vi "get_mlt.vi"   [LabVIEW 2012]
uses:
  <vilib>/addons/internet/NI_InternetTK_Core_VIs.lvlib
types:
  T1 = typedef "CGI Connection Info.ctl" = cluster{"name":string, "type":T2, "session":T3}
  T2 = typedef "CGI Request Type.ctl" = enum16{"cgi", ".spool first", ".spool", ".spool last"}
  T3 = typedef "HTTP Session.ctl" = refnum<k1>
  T4 = typedef "NI_FTP.lvlib/Keyed Array.ctl" = cluster{"keys":string[], "values":string[]}
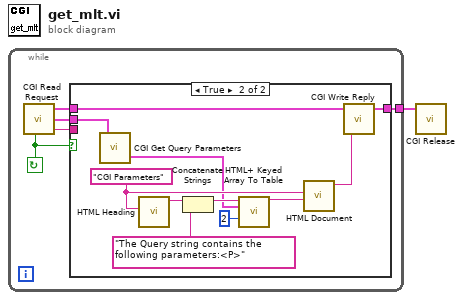
[diagram p0: block diagram]
diagram:
  n1 = while {
    tunnel: [w5] -> w1
    stop <- w4 continue-if-true
    n2 = call <vilib>:"CGI Read Request.vi"() -> ("valid request?"=w4:bool, "cgi connection info"=w6:T1, "env"=w3:T4, "content"=w2:string)  [unwired: 4 in]
    n3 = case shown="True" w4 {
      tunnel: [w7 w18] -> w5
      tunnel: w6 -> [w7 w17]
      tunnel: w3 -> [_ w15]
      tunnel: w2 -> [_ _]
      frame False {
      }
      frame True {
        w14 = "CGI Parameters" ("heading")
        n4 = call <vilib>:"CGI Get Query Parameters.vi"("env"=w15) -> ("query params"=w10:T4)  [unwired: 2 out]
        n5 = call <vilib>:"HTML Heading.vi"("heading"=w14) -> ("HTML out"=w13:string)  [unwired: 10 in]
        n6 = Concatenate Strings(w13, "The Query string contains the following parameters:<P>" ("label")) -> (w12:string)
        n7 = call <vilib>:"HTML+ Keyed Array To Table.vi"("HTML in"=w12, "keyed array"=w10, "border width (default)"=2) -> ("HTML out"=w9:string)  [unwired: 12 in]
        n8 = call <vilib>:"HTML Document.vi"("document body"=w9, "document title"=w14) -> ("HTML Document"=w16:string)  [unwired: 9 in]
        n9 = call <vilib>:"CGI Write Reply.vi"("content"=w16, "cgi connection info"=w17) -> ("cgi connection info out"=w18:T1)  [unwired: 3 in]
      }
    }
  }
  n10 = call <vilib>:"CGI Release.vi"("cgi connection info"=w1) -> ()  [unwired: 5 in]
